vi "next.vi"(8 "error in (no error)":errorcluster, 11 "NameIterator in":refnum<class "NameIterator.lvclass">) -> (0 "error out":errorcluster, 2 "Name":string, 3 "NameIterator out":refnum<class "NameIterator.lvclass">)   [LabVIEW 2016, in "NameIterator.lvclass"]
uses:
  NameIterator.lvclass
  NameIterator.lvclass/NameIterator.ctl
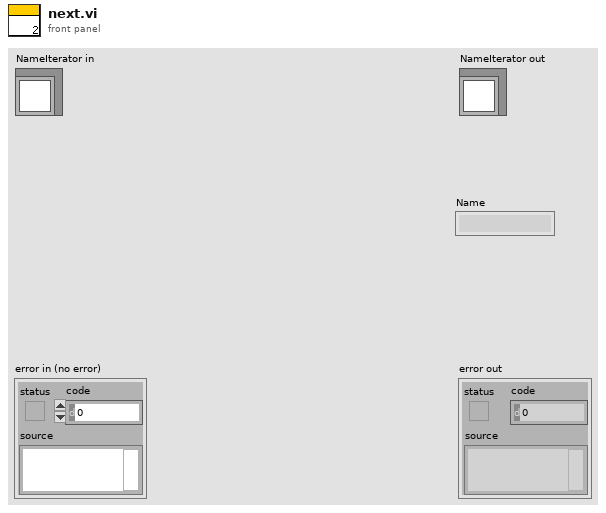
[diagram p1: front panel]
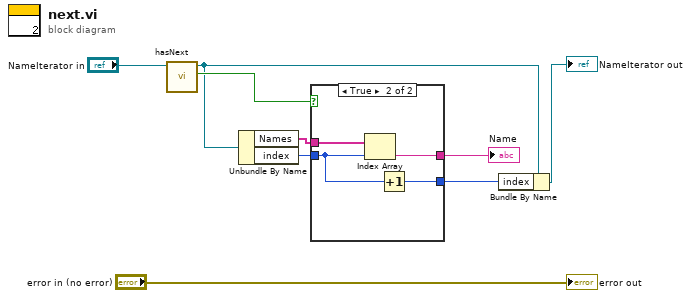
[diagram p0: block diagram]
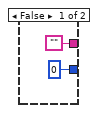
[diagram p2: hidden frame]
diagram:
  n1 = call-dynamic "hasNext.vi"("NameIterator in"="NameIterator in") -> ("hasNext?"=w8:bool, "NameIterator out"=w2:refnum<class "NameIterator.lvclass">)  [unwired: 8 in, 1 out]
  n2 = Unbundle By Name(w2) -> ("Names"=w1:string[], "index"=w6:i32)
  n3 = case shown="True" w8 {
    tunnel: w6 -> [_ w14]
    tunnel: w1 -> [_ w15]
    tunnel: [0 w12] -> w4
    tunnel: ["" w13] -> w5
    frame False {
    }
    frame True {
      n4 = Index Array(array=w15, index=w14) -> (element=w13:string)
      n5 = Increment(x=w14) -> (x+1=w12:i32)
    }
  }
  "Name" <- w5
  n6 = Bundle By Name(cluster=w2, "index"=w4) -> (→"NameIterator out":refnum<class "NameIterator.lvclass">)
  "error out" <- "error in (no error)"
